vi "Lab Panel V5.26.vi"() -> ()   [LabVIEW 2017] (continued)
                                n855 = TDMS Open(6:FALSE, 10:T21."create or replace" ("operation (0:open)"), 11:w1499) -> (0:w1498:errorcluster, 3:→"TDMS LAB03-2":refnum<k34>)  [unwired: 4 in]
                              }
                              frame #2 {
                                n856 = local read "SET LAB03-2"() -> (w1509:T5)
                                n857 = local read "TDMS LAB03-2"() -> (w1520:refnum<k34>)
                                n858 = Build Array("Testers Name", "Description", "Set Test Cycles", "T-Rise minutes", "T-Rise Deg C") -> (w1510:string[])
                                n859 = Unbundle(w1509) -> ("NAME"=w1508:string, "DESCRIPTION"=w1507:string, "CYCLES"=w1506:dbl, "T-RISE mins"=w1505:dbl, "T-RISE deg C"=w1504:dbl)
                                n860 = Number To Decimal String(number=w1506) -> (decimal integer string=w1519:string)  [unwired: 1 in]
                                n861 = Number To Decimal String(number=w1505) -> (decimal integer string=w1518:string)  [unwired: 1 in]
                                n862 = Number To Decimal String(number=w1504) -> (decimal integer string=w1517:string)  [unwired: 1 in]
                                n863 = Build Array(w1508, w1507, w1519, w1518, w1517) -> (w1516:string[])
                                n864 = TDMS Set Properties(5:w1516, 7:w1510, 11:w1520) -> ()  [unwired: 3 in, 4 out]
                              }
                              frame #3 {
                                n865 = local read "DISP LAB03-2"() -> (w1525:T4)
                                n866 = Concatenate Strings("LAB03-2  ", w1524) -> (w1526:string)
                                n867 = Two Button Dialog(message=w1526, 1:w1522, 2:w1523) -> (T button?=w1528:bool)
                                n868 = case shown="True" w1528 {
                                tunnel: w1525 -> [w1535 w1536]
                                tunnel: [w1535 w1536] -> w1532
                                tunnel: [w1534 w1537] -> w1531
                                tunnel: [w1533 w1537] -> w1530
                                frame False {
                                n869 = Unbundle(w1535) -> ("CYCLE"=w1534:dbl, "MINS"=w1533:dbl)  [unwired: 1 out]
                                }
                                frame True {
                                w1537 = 0.0
                                }
                                }
                                n870 = Bundle(cluster=w1532, "CYCLE"=w1531, "MINS"=w1530, "STATUS"="RUN") -> (w1521:T4)
                                n871 = local write "DISP LAB03-2"(w1521) -> ()
                              }
                              frame #4 {
                                n872 = local read "TEMP START LAB03-2"() -> (w1540:cluster{"TL":dbl, "TN":dbl})
                                n873 = Bundle(cluster=w1540, "TL"=w1538, "TN"=w1538) -> (w1539:cluster{"TL":dbl, "TN":dbl})
                                n874 = local write "TEMP START LAB03-2"(w1539) -> ()
                              }
                            }
                          }
                        }
                      }
                    }
                  }
                }
              }
              event "RUN LAB04-1": Value Change {
                n875 = event-data() -> ("NewVal"=w1545:bool)  [unwired: 1 in, 5 out]
                n876 = local write "run lab04-1"(w1545) -> ()
                n877 = case shown="True" w1545 {
                  tunnel: w1551 -> [_ w1589]
                  tunnel: w1550 -> [_ w1588]
                  tunnel: w1548 -> [w1553 w1587]
                  tunnel: w1549 -> [_ w1586]
                  tunnel: w1547 -> [_ w1585]
                  tunnel: [w1552 w1584] -> w1546
                  tunnel: w1544 -> [_ w1583]
                  tunnel: w1543 -> [_ w1582]
                  tunnel: w1542 -> [_ w1581]
                  tunnel: w1541 -> [_ w1579]
                  frame False {
                    # "stop test"
                    n878 = stacked-sequence {
                      tunnel: w1553 -> [w1562 _]
                      tunnel: [w1554 _] -> w1552
                      frame #0 {
                        n879 = local read "DISP LAB04-1"() -> (w1561:T4)
                        n880 = Unbundle(w1561) -> ("CYCLE"=w1559:dbl, "MINS"=w1560:dbl)  [unwired: 1 out]
                        n881 = case shown="\"CYCLE TEST\"" w1562 {
                          tunnel: w1560 -> [_ _ w1569]
                          tunnel: w1559 -> [w1567 w1568 _]
                          tunnel: [w1567 w1568 w1569] -> w1558
                          frame "CHART TEST", Default {
                          }
                          frame "CYCLE TEST" {
                          }
                          frame "T-RISE TEST" {
                          }
                        }
                        n882 = local read "TDMS LAB04-1"() -> (w1566:refnum<k34>)
                        n883 = Build Array("STOPPED") -> (w1563:string[])
                        n884 = Build Array(w1558) -> (w1557:dbl[])
                        n885 = TDMS Write(0:w1566, 5:"TEST RESULT", 7:w1563, 9:w1557) -> (4:w1555:refnum<k34>, 15:w1556:errorcluster)  [unwired: 2 in, 2 out]
                        n886 = TDMS Close(8:w1556, 11:w1555) -> (0:w1554:errorcluster)  [unwired: 1 out]
                      }
                      frame #1 {
                        n887 = local read "DISP LAB04-1"() -> (w1573:T4)
                        n888 = stacked-sequence {
                          tunnel: "LAB04-1" -> [w1575 w1577]
                          frame #0 {
                            n889 = call "sub vi - defrag tdms v1.vi"("panel id"=w1575) -> ("error out"=w1574:errorcluster)  [unwired: 10 in]
                            n890 = local write "data file error"(w1574) -> ()
                          }
                          frame #1 {
                            n891 = call "Save data file (stop) v3.vi"("panel id"=w1577) -> ("network file save error"=w1576:errorcluster)  [unwired: 9 in, 1 out]
                            n892 = local write "RESULT LAB04-1"(FALSE) -> ()
                            n893 = local write "data file error"(w1576) -> ()
                          }
                        }
                        n894 = Bundle(cluster=w1573, "STATUS"="STOP") -> (w1571:T4)  [unwired: 2 in]
                        n895 = local write "DISP LAB04-1"(w1571) -> ()
                      }
                    }
                  }
                  frame True {
                    n896 = local read "SIG LAB04-1"() -> (w1580:T2)
                    n897 = stacked-sequence {
                      seq-local: [w1591 _] -> [_ w1595]
                      tunnel: w1589 -> [_ w1605]
                      tunnel: w1588 -> [_ w1604]
                      tunnel: w1587 -> [_ w1603]
                      tunnel: w1586 -> [_ w1602]
                      tunnel: w1585 -> [_ w1601]
                      tunnel: [_ w1600] -> w1584
                      tunnel: w1583 -> [_ w1599]
                      tunnel: w1582 -> [_ w1598]
                      tunnel: w1581 -> [_ w1597]
                      tunnel: w1580 -> [w1590 w1596]
                      tunnel: w1579 -> [_ w1594]
                      frame #0 {
                        n898 = Unbundle(w1590) -> ("AMPS"=w1593:dbl)  [unwired: 4 out]
                        n899 = call "Check For Amps on v1.vi"("ID"="LAB04-1", "amps"=w1593) -> ("amps"=w1591:bool)  [unwired: 9 in]
                      }
                      frame #1 {
                        n900 = case shown="True" w1595 {
                          tunnel: w1605 -> [_ w1618]
                          tunnel: w1604 -> [_ w1617]
                          tunnel: w1603 -> [_ w1616]
                          tunnel: w1602 -> [_ w1615]
                          tunnel: w1601 -> [_ w1614]
                          tunnel: [errorcluster {"status"=FALSE, "code"=0, "source"=""} ("error out") w1613] -> w1600
                          tunnel: w1599 -> [_ w1612]
                          tunnel: w1598 -> [_ w1611]
                          tunnel: w1597 -> [_ w1610]
                          tunnel: w1596 -> [_ w1609]
                          tunnel: w1594 -> [_ w1608]
                          frame False {
                            w1606 = FALSE
                            n901 = local write "RUN LAB04-1"(w1606) -> ()
                            n902 = local write "run lab04-1"(w1606) -> ()
                          }
                          frame True {
                            n903 = stacked-sequence {
                              seq-local: [w1619 _ _ _ _] -> [_ w1643 _ _ _]
                              tunnel: w1618 -> [w1624 _ _ _ _]
                              tunnel: w1617 -> [w1620 _ _ _ _]
                              tunnel: w1616 -> [w1634 _ _ _ _]
                              tunnel: w1615 -> [w1627 _ _ _ _]
                              tunnel: w1614 -> [w1622 _ _ _ _]
                              tunnel: [_ w1638 _ _ _] -> w1613
                              tunnel: w1612 -> [_ _ _ w1664 _]
                              tunnel: w1611 -> [_ _ _ w1663 _]
                              tunnel: w1610 -> [_ _ _ w1662 _]
                              tunnel: w1609 -> [_ _ _ _ _]
                              tunnel: w1608 -> [_ _ _ _ w1678]
                              frame #0 {
                                w1621 = "\\"
                                n904 = local read "SET LAB04-1"() -> (w1629:T5)
                                n905 = case shown="\"CYCLE TEST\"" w1634 {
                                tunnel: ["L04-1-CHART TEST-" "L04-1-CYCLE TEST-" "L04-1-T-RISE TEST-"] -> w1630
                                frame "CHART TEST", Default {
                                }
                                frame "CYCLE TEST" {
                                }
                                frame "T-RISE TEST" {
                                }
                                }
                                n906 = Unbundle(w1629) -> ("DESCRIPTION"=w1628:string)  [unwired: 4 out]
                                n907 = Concatenate Strings(w1624, "\\", w1622, w1621, w1620, w1621) -> (w1631:string)
                                n908 = String To Path(string=w1631) -> (path=w1633:path)
                                n909 = Concatenate Strings(w1631, w1630, w1628, "-", w1627, ".tdms") -> (w1619:string)
                                n910 = Create Folder(path (use dialog)=w1633) -> (error out=w1632:errorcluster)  [unwired: 2 in, 2 out]
                                n911 = global write "Global 1.vi" "LAB04-1 FILE"(w1619) -> ()
                                n912 = call <vilib>:"Clear Errors.vi"("error in (no error)"=w1632) -> ()  [unwired: 5 in, 2 out]
                              }
                              frame #1 {
                                (unwired) FALSE
                                n913 = String To Path(string=w1643) -> (path=w1639:path)
                                n914 = TDMS Open(6:FALSE, 10:T21."create or replace" ("operation (0:open)"), 11:w1639) -> (0:w1638:errorcluster, 3:→"TDMS LAB04-1":refnum<k34>)  [unwired: 4 in]
                              }
                              frame #2 {
                                n915 = local read "SET LAB04-1"() -> (w1649:T5)
                                n916 = local read "TDMS LAB04-1"() -> (w1660:refnum<k34>)
                                n917 = Build Array("Testers Name", "Description", "Set Test Cycles", "T-Rise minutes", "T-Rise Deg C") -> (w1650:string[])
                                n918 = Unbundle(w1649) -> ("NAME"=w1648:string, "DESCRIPTION"=w1647:string, "CYCLES"=w1646:dbl, "T-RISE mins"=w1645:dbl, "T-RISE deg C"=w1644:dbl)
                                n919 = Number To Decimal String(number=w1646) -> (decimal integer string=w1659:string)  [unwired: 1 in]
                                n920 = Number To Decimal String(number=w1645) -> (decimal integer string=w1658:string)  [unwired: 1 in]
                                n921 = Number To Decimal String(number=w1644) -> (decimal integer string=w1657:string)  [unwired: 1 in]
                                n922 = Build Array(w1648, w1647, w1659, w1658, w1657) -> (w1656:string[])
                                n923 = TDMS Set Properties(5:w1656, 7:w1650, 11:w1660) -> ()  [unwired: 3 in, 4 out]
                              }
                              frame #3 {
                                n924 = local read "DISP LAB04-1"() -> (w1665:T4)
                                n925 = Concatenate Strings("LAB04-1  ", w1664) -> (w1666:string)
                                n926 = Two Button Dialog(message=w1666, 1:w1662, 2:w1663) -> (T button?=w1668:bool)
                                n927 = case shown="True" w1668 {
                                tunnel: w1665 -> [w1675 w1676]
                                tunnel: [w1675 w1676] -> w1672
                                tunnel: [w1674 w1677] -> w1671
                                tunnel: [w1673 w1677] -> w1670
                                frame False {
                                n928 = Unbundle(w1675) -> ("CYCLE"=w1674:dbl, "MINS"=w1673:dbl)  [unwired: 1 out]
                                }
                                frame True {
                                w1677 = 0.0
                                }
                                }
                                n929 = Bundle(cluster=w1672, "CYCLE"=w1671, "MINS"=w1670, "STATUS"="RUN") -> (w1661:T4)
                                n930 = local write "DISP LAB04-1"(w1661) -> ()
                              }
                              frame #4 {
                                n931 = local read "TEMP START LAB04-1"() -> (w1680:cluster{"TL":dbl, "TN":dbl})
                                n932 = Bundle(cluster=w1680, "TL"=w1678, "TN"=w1678) -> (w1679:cluster{"TL":dbl, "TN":dbl})
                                n933 = local write "TEMP START LAB04-1"(w1679) -> ()
                              }
                            }
                          }
                        }
                      }
                    }
                  }
                }
              }
              event "RUN LAB04-2": Value Change {
                n934 = event-data() -> ("NewVal"=w1685:bool)  [unwired: 1 in, 5 out]
                n935 = local write "run lab04-2"(w1685) -> ()
                n936 = case shown="True" w1685 {
                  tunnel: w1691 -> [_ w1729]
                  tunnel: w1690 -> [_ w1728]
                  tunnel: w1688 -> [w1693 w1727]
                  tunnel: w1689 -> [_ w1726]
                  tunnel: w1687 -> [_ w1725]
                  tunnel: [w1692 w1724] -> w1686
                  tunnel: w1684 -> [_ w1723]
                  tunnel: w1683 -> [_ w1722]
                  tunnel: w1682 -> [_ w1721]
                  tunnel: w1681 -> [_ w1719]
                  frame False {
                    # "stop test"
                    n937 = stacked-sequence {
                      tunnel: w1693 -> [w1702 _]
                      tunnel: [w1694 _] -> w1692
                      frame #0 {
                        n938 = local read "DISP LAB04-2"() -> (w1701:T4)
                        n939 = Unbundle(w1701) -> ("CYCLE"=w1699:dbl, "MINS"=w1700:dbl)  [unwired: 1 out]
                        n940 = case shown="\"CYCLE TEST\"" w1702 {
                          tunnel: w1700 -> [_ _ w1709]
                          tunnel: w1699 -> [w1707 w1708 _]
                          tunnel: [w1707 w1708 w1709] -> w1698
                          frame "CHART TEST", Default {
                          }
                          frame "CYCLE TEST" {
                          }
                          frame "T-RISE TEST" {
                          }
                        }
                        n941 = local read "TDMS LAB04-2"() -> (w1706:refnum<k34>)
                        n942 = Build Array("STOPPED") -> (w1703:string[])
                        n943 = Build Array(w1698) -> (w1697:dbl[])
                        n944 = TDMS Write(0:w1706, 5:"TEST RESULT", 7:w1703, 9:w1697) -> (4:w1695:refnum<k34>, 15:w1696:errorcluster)  [unwired: 2 in, 2 out]
                        n945 = TDMS Close(8:w1696, 11:w1695) -> (0:w1694:errorcluster)  [unwired: 1 out]
                      }
                      frame #1 {
                        n946 = local read "DISP LAB04-2"() -> (w1713:T4)
                        n947 = stacked-sequence {
                          tunnel: "LAB04-2" -> [w1715 w1717]
                          frame #0 {
                            n948 = call "sub vi - defrag tdms v1.vi"("panel id"=w1715) -> ("error out"=w1714:errorcluster)  [unwired: 10 in]
                            n949 = local write "data file error"(w1714) -> ()
                          }
                          frame #1 {
                            n950 = call "Save data file (stop) v3.vi"("panel id"=w1717) -> ("network file save error"=w1716:errorcluster)  [unwired: 9 in, 1 out]
                            n951 = local write "RESULT LAB04-2"(FALSE) -> ()
                            n952 = local write "data file error"(w1716) -> ()
                          }
                        }
                        n953 = Bundle(cluster=w1713, "STATUS"="STOP") -> (w1711:T4)  [unwired: 2 in]
                        n954 = local write "DISP LAB04-2"(w1711) -> ()
                      }
                    }
                  }
                  frame True {
                    n955 = local read "SIG LAB04-2"() -> (w1720:T2)
                    n956 = stacked-sequence {
                      seq-local: [w1731 _] -> [_ w1735]
                      tunnel: w1729 -> [_ w1745]
                      tunnel: w1728 -> [_ w1744]
                      tunnel: w1727 -> [_ w1743]
                      tunnel: w1726 -> [_ w1742]
                      tunnel: w1725 -> [_ w1741]
                      tunnel: [_ w1740] -> w1724
                      tunnel: w1723 -> [_ w1739]
                      tunnel: w1722 -> [_ w1738]
                      tunnel: w1721 -> [_ w1737]
                      tunnel: w1720 -> [w1730 w1736]
                      tunnel: w1719 -> [_ w1734]
                      frame #0 {
                        n957 = Unbundle(w1730) -> ("AMPS"=w1733:dbl)  [unwired: 4 out]
                        n958 = call "Check For Amps on v1.vi"("ID"="LAB04-2", "amps"=w1733) -> ("amps"=w1731:bool)  [unwired: 9 in]
                      }
                      frame #1 {
                        n959 = case shown="True" w1735 {
                          tunnel: w1745 -> [_ w1758]
                          tunnel: w1744 -> [_ w1757]
                          tunnel: w1743 -> [_ w1756]
                          tunnel: w1742 -> [_ w1755]
                          tunnel: w1741 -> [_ w1754]
                          tunnel: [errorcluster {"status"=FALSE, "code"=0, "source"=""} ("error out") w1753] -> w1740
                          tunnel: w1739 -> [_ w1752]
                          tunnel: w1738 -> [_ w1751]
                          tunnel: w1737 -> [_ w1750]
                          tunnel: w1736 -> [_ w1749]
                          tunnel: w1734 -> [_ w1748]
                          frame False {
                            w1746 = FALSE
                            n960 = local write "RUN LAB04-2"(w1746) -> ()
                            n961 = local write "run lab04-2"(w1746) -> ()
                          }
                          frame True {
                            n962 = stacked-sequence {
                              seq-local: [w1759 _ _ _ _] -> [_ w1783 _ _ _]
                              tunnel: w1758 -> [w1764 _ _ _ _]
                              tunnel: w1757 -> [w1760 _ _ _ _]
                              tunnel: w1756 -> [w1774 _ _ _ _]
                              tunnel: w1755 -> [w1767 _ _ _ _]
                              tunnel: w1754 -> [w1762 _ _ _ _]
                              tunnel: [_ w1778 _ _ _] -> w1753
                              tunnel: w1752 -> [_ _ _ w1804 _]
                              tunnel: w1751 -> [_ _ _ w1803 _]
                              tunnel: w1750 -> [_ _ _ w1802 _]
                              tunnel: w1749 -> [_ _ _ _ _]
                              tunnel: w1748 -> [_ _ _ _ w1818]
                              frame #0 {
                                w1761 = "\\"
                                n963 = local read "SET LAB04-2"() -> (w1769:T5)
                                n964 = case shown="\"CHART TEST\", Default" w1774 {
                                tunnel: ["L04-2-CHART TEST-" "L04-2-CYCLE TEST-" "L04-2-T-RISE TEST-"] -> w1770
                                frame "CHART TEST", Default {
                                }
                                frame "CYCLE TEST" {
                                }
                                frame "T-RISE TEST" {
                                }
                                }
                                n965 = Unbundle(w1769) -> ("DESCRIPTION"=w1768:string)  [unwired: 4 out]
                                n966 = Concatenate Strings(w1764, "\\", w1762, w1761, w1760, w1761) -> (w1771:string)
                                n967 = String To Path(string=w1771) -> (path=w1773:path)
                                n968 = Concatenate Strings(w1771, w1770, w1768, "-", w1767, ".tdms") -> (w1759:string)
                                n969 = Create Folder(path (use dialog)=w1773) -> (error out=w1772:errorcluster)  [unwired: 2 in, 2 out]
                                n970 = global write "Global 1.vi" "LAB04-2 FILE"(w1759) -> ()
                                n971 = call <vilib>:"Clear Errors.vi"("error in (no error)"=w1772) -> ()  [unwired: 5 in, 2 out]
                              }
                              frame #1 {
                                (unwired) FALSE
                                n972 = String To Path(string=w1783) -> (path=w1779:path)
                                n973 = TDMS Open(6:FALSE, 10:T21."create or replace" ("operation (0:open)"), 11:w1779) -> (0:w1778:errorcluster, 3:→"TDMS LAB04-2":refnum<k34>)  [unwired: 4 in]
                              }
                              frame #2 {
                                n974 = local read "SET LAB04-2"() -> (w1789:T5)
                                n975 = local read "TDMS LAB04-2"() -> (w1800:refnum<k34>)
                                n976 = Build Array("Testers Name", "Description", "Set Test Cycles", "T-Rise minutes", "T-Rise Deg C") -> (w1790:string[])
                                n977 = Unbundle(w1789) -> ("NAME"=w1788:string, "DESCRIPTION"=w1787:string, "CYCLES"=w1786:dbl, "T-RISE mins"=w1785:dbl, "T-RISE deg C"=w1784:dbl)
                                n978 = Number To Decimal String(number=w1786) -> (decimal integer string=w1799:string)  [unwired: 1 in]
                                n979 = Number To Decimal String(number=w1785) -> (decimal integer string=w1798:string)  [unwired: 1 in]
                                n980 = Number To Decimal String(number=w1784) -> (decimal integer string=w1797:string)  [unwired: 1 in]
                                n981 = Build Array(w1788, w1787, w1799, w1798, w1797) -> (w1796:string[])
                                n982 = TDMS Set Properties(5:w1796, 7:w1790, 11:w1800) -> ()  [unwired: 3 in, 4 out]
                              }
                              frame #3 {
                                n983 = local read "DISP LAB04-2"() -> (w1805:T4)
                                n984 = Concatenate Strings("LAB04-2 ", w1804) -> (w1806:string)
                                n985 = Two Button Dialog(message=w1806, 1:w1802, 2:w1803) -> (T button?=w1808:bool)
                                n986 = case shown="True" w1808 {
                                tunnel: w1805 -> [w1815 w1816]
                                tunnel: [w1815 w1816] -> w1812
                                tunnel: [w1814 w1817] -> w1811
                                tunnel: [w1813 w1817] -> w1810
                                frame False {
                                n987 = Unbundle(w1815) -> ("CYCLE"=w1814:dbl, "MINS"=w1813:dbl)  [unwired: 1 out]
                                }
                                frame True {
                                w1817 = 0.0
                                }
                                }
                                n988 = Bundle(cluster=w1812, "CYCLE"=w1811, "MINS"=w1810, "STATUS"="RUN") -> (w1801:T4)
                                n989 = local write "DISP LAB04-2"(w1801) -> ()
                              }
                              frame #4 {
                                n990 = local read "TEMP START LAB04-2"() -> (w1820:cluster{"TL":dbl, "TN":dbl})
                                n991 = Bundle(cluster=w1820, "TL"=w1818, "TN"=w1818) -> (w1819:cluster{"TL":dbl, "TN":dbl})
                                n992 = local write "TEMP START LAB04-2"(w1819) -> ()
                              }
                            }
                          }
                        }
                      }
                    }
                  }
                }
              }
              event "RUN LAB05-1": Value Change {
                n993 = event-data() -> ("NewVal"=w1825:bool)  [unwired: 1 in, 5 out]
                n994 = local write "run lab05-1"(w1825) -> ()
                n995 = case shown="True" w1825 {
                  tunnel: w1831 -> [_ w1869]
                  tunnel: w1830 -> [_ w1868]
                  tunnel: w1828 -> [w1833 w1867]
                  tunnel: w1829 -> [_ w1866]
                  tunnel: w1827 -> [_ w1865]
                  tunnel: [w1832 w1864] -> w1826
                  tunnel: w1824 -> [_ w1863]
                  tunnel: w1823 -> [_ w1862]
                  tunnel: w1822 -> [_ w1861]
                  tunnel: w1821 -> [_ w1859]
                  frame False {
                    # "stop test"
                    n996 = stacked-sequence {
                      tunnel: w1833 -> [w1842 _]
                      tunnel: [w1834 _] -> w1832
                      frame #0 {
                        n997 = local read "DISP LAB05-1"() -> (w1841:T4)
                        n998 = Unbundle(w1841) -> ("CYCLE"=w1839:dbl, "MINS"=w1840:dbl)  [unwired: 1 out]
                        n999 = case shown="\"CYCLE TEST\"" w1842 {
                          tunnel: w1840 -> [_ _ w1849]
                          tunnel: w1839 -> [w1847 w1848 _]
                          tunnel: [w1847 w1848 w1849] -> w1838
                          frame "CHART TEST", Default {
                          }
                          frame "CYCLE TEST" {
                          }
                          frame "T-RISE TEST" {
                          }
                        }
                        n1000 = local read "TDMS LAB05-1"() -> (w1846:refnum<k34>)
                        n1001 = Build Array("STOPPED") -> (w1843:string[])
                        n1002 = Build Array(w1838) -> (w1837:dbl[])
                        n1003 = TDMS Write(0:w1846, 5:"TEST RESULT", 7:w1843, 9:w1837) -> (4:w1835:refnum<k34>, 15:w1836:errorcluster)  [unwired: 2 in, 2 out]
                        n1004 = TDMS Close(8:w1836, 11:w1835) -> (0:w1834:errorcluster)  [unwired: 1 out]
                      }
                      frame #1 {
                        n1005 = local read "DISP LAB05-1"() -> (w1853:T4)
                        n1006 = stacked-sequence {
                          tunnel: "LAB05-1" -> [w1855 w1857]
                          frame #0 {
                            n1007 = call "sub vi - defrag tdms v1.vi"("panel id"=w1855) -> ("error out"=w1854:errorcluster)  [unwired: 10 in]
                            n1008 = local write "data file error"(w1854) -> ()
                          }
                          frame #1 {
                            n1009 = call "Save data file (stop) v3.vi"("panel id"=w1857) -> ("network file save error"=w1856:errorcluster)  [unwired: 9 in, 1 out]
                            n1010 = local write "RESULT LAB05-1"(FALSE) -> ()
                            n1011 = local write "data file error"(w1856) -> ()
                          }
                        }
                        n1012 = Bundle(cluster=w1853, "STATUS"="STOP") -> (w1851:T4)  [unwired: 2 in]
                        n1013 = local write "DISP LAB05-1"(w1851) -> ()
                      }
                    }
                  }
                  frame True {
                    n1014 = local read "SIG LAB05-1"() -> (w1860:T2)
                    n1015 = stacked-sequence {
                      seq-local: [w1871 _] -> [_ w1875]
                      tunnel: w1869 -> [_ w1885]
                      tunnel: w1868 -> [_ w1884]
                      tunnel: w1867 -> [_ w1883]
                      tunnel: w1866 -> [_ w1882]
                      tunnel: w1865 -> [_ w1881]
                      tunnel: [_ w1880] -> w1864
                      tunnel: w1863 -> [_ w1879]
                      tunnel: w1862 -> [_ w1878]
                      tunnel: w1861 -> [_ w1877]
                      tunnel: w1860 -> [w1870 w1876]
                      tunnel: w1859 -> [_ w1874]
                      frame #0 {
                        n1016 = Unbundle(w1870) -> ("AMPS"=w1873:dbl)  [unwired: 4 out]
                        n1017 = call "Check For Amps on v1.vi"("ID"="LAB05-1", "amps"=w1873) -> ("amps"=w1871:bool)  [unwired: 9 in]
                      }
                      frame #1 {
                        n1018 = case shown="True" w1875 {
                          tunnel: w1885 -> [_ w1898]
                          tunnel: w1884 -> [_ w1897]
                          tunnel: w1883 -> [_ w1896]
                          tunnel: w1882 -> [_ w1895]
                          tunnel: w1881 -> [_ w1894]
                          tunnel: [errorcluster {"status"=FALSE, "code"=0, "source"=""} ("error out") w1893] -> w1880
                          tunnel: w1879 -> [_ w1892]
                          tunnel: w1878 -> [_ w1891]
                          tunnel: w1877 -> [_ w1890]
                          tunnel: w1876 -> [_ w1889]
                          tunnel: w1874 -> [_ w1888]
                          frame False {
                            w1886 = FALSE
                            n1019 = local write "RUN LAB05-1"(w1886) -> ()
                            n1020 = local write "run lab05-1"(w1886) -> ()
                          }
                          frame True {
                            n1021 = stacked-sequence {
                              seq-local: [w1899 _ _ _ _] -> [_ w1923 _ _ _]
                              tunnel: w1898 -> [w1904 _ _ _ _]
                              tunnel: w1897 -> [w1900 _ _ _ _]
                              tunnel: w1896 -> [w1914 _ _ _ _]
                              tunnel: w1895 -> [w1907 _ _ _ _]
                              tunnel: w1894 -> [w1902 _ _ _ _]
                              tunnel: [_ w1918 _ _ _] -> w1893
                              tunnel: w1892 -> [_ _ _ w1943 _]
                              tunnel: w1891 -> [_ _ _ w1942 _]
                              tunnel: w1890 -> [_ _ _ w1941 _]
                              tunnel: w1889 -> [_ _ _ _ _]
                              tunnel: w1888 -> [_ _ _ _ w1958]
                              frame #0 {
                                w1901 = "\\"
                                n1022 = local read "SET LAB05-1"() -> (w1909:T5)
                                n1023 = case shown="\"CYCLE TEST\"" w1914 {
                                tunnel: ["L05-1-CHART TEST-" "L05-1-CYCLE TEST-" "L05-1-T-RISE TEST-"] -> w1910
                                frame "CHART TEST", Default {
                                }
                                frame "CYCLE TEST" {
                                }
                                frame "T-RISE TEST" {
                                }
                                }
                                n1024 = Unbundle(w1909) -> ("DESCRIPTION"=w1908:string)  [unwired: 4 out]
                                n1025 = Concatenate Strings(w1904, "\\", w1902, w1901, w1900, w1901) -> (w1911:string)
                                n1026 = String To Path(string=w1911) -> (path=w1913:path)
                                n1027 = Concatenate Strings(w1911, w1910, w1908, "-", w1907, ".tdms") -> (w1899:string)
                                n1028 = Create Folder(path (use dialog)=w1913) -> (error out=w1912:errorcluster)  [unwired: 2 in, 2 out]
                                n1029 = global write "Global 1.vi" "LAB05-1 FILE"(w1899) -> ()
                                n1030 = call <vilib>:"Clear Errors.vi"("error in (no error)"=w1912) -> ()  [unwired: 5 in, 2 out]
                              }
                              frame #1 {
                                (unwired) FALSE
                                n1031 = String To Path(string=w1923) -> (path=w1919:path)
                                n1032 = TDMS Open(6:FALSE, 10:T21."create or replace" ("operation (0:open)"), 11:w1919) -> (0:w1918:errorcluster, 3:→"TDMS LAB05-1":refnum<k34>)  [unwired: 4 in]
                              }
                              frame #2 {
                                n1033 = local read "SET LAB05-1"() -> (w1929:T5)
                                n1034 = local read "TDMS LAB05-1"() -> (w1940:refnum<k34>)
                                n1035 = Build Array("Testers Name", "Description", "Set Test Cycles", "T-Rise minutes", "T-Rise Deg C") -> (w1930:string[])
                                n1036 = Unbundle(w1929) -> ("NAME"=w1928:string, "DESCRIPTION"=w1927:string, "CYCLES"=w1926:dbl, "T-RISE mins"=w1925:dbl, "T-RISE deg C"=w1924:dbl)
                                n1037 = Number To Decimal String(number=w1926) -> (decimal integer string=w1939:string)  [unwired: 1 in]
                                n1038 = Number To Decimal String(number=w1925) -> (decimal integer string=w1938:string)  [unwired: 1 in]
                                n1039 = Number To Decimal String(number=w1924) -> (decimal integer string=w1937:string)  [unwired: 1 in]
                                n1040 = Build Array(w1928, w1927, w1939, w1938, w1937) -> (w1936:string[])
                                n1041 = TDMS Set Properties(5:w1936, 7:w1930, 11:w1940) -> ()  [unwired: 3 in, 4 out]
                              }
                              frame #3 {
                                n1042 = local read "DISP LAB05-1"() -> (w1945:T4)
                                n1043 = Concatenate Strings("LAB05-1  ", w1943) -> (w1946:string)
                                n1044 = Two Button Dialog(message=w1946, 1:w1941, 2:w1942) -> (T button?=w1948:bool)
                                n1045 = case shown="True" w1948 {
                                tunnel: w1945 -> [w1955 w1956]
                                tunnel: [w1955 w1956] -> w1952
                                tunnel: [w1954 w1957] -> w1951
                                tunnel: [w1953 w1957] -> w1950
                                frame False {
                                n1046 = Unbundle(w1955) -> ("CYCLE"=w1954:dbl, "MINS"=w1953:dbl)  [unwired: 1 out]
                                }
                                frame True {
                                w1957 = 0.0
                                }
                                }
                                n1047 = Bundle(cluster=w1952, "CYCLE"=w1951, "MINS"=w1950, "STATUS"="RUN") -> (w1944:T4)
                                n1048 = local write "DISP LAB05-1"(w1944) -> ()
                              }
                              frame #4 {
                                n1049 = local read "TEMP START LAB05-1"() -> (w1960:cluster{"TL":dbl, "TN":dbl})
                                n1050 = Bundle(cluster=w1960, "TL"=w1958, "TN"=w1958) -> (w1959:cluster{"TL":dbl, "TN":dbl})
                                n1051 = local write "TEMP START LAB05-1"(w1959) -> ()
                              }
                            }
                          }
                        }
                      }
                    }
                  }
                }
              }
              event "RUN LAB05-2": Value Change {
                n1052 = event-data() -> ("NewVal"=w1966:bool)  [unwired: 1 in, 5 out]
                n1053 = local read "SIG LAB05-2"() -> (w1962:T2)
                n1054 = case shown="True" w1966 {
                  tunnel: w1972 -> [_ w2010]
                  tunnel: w1971 -> [_ w2009]
                  tunnel: w1969 -> [w1974 w2008]
                  tunnel: w1970 -> [_ w2007]
                  tunnel: w1968 -> [_ w2006]
                  tunnel: [w1973 w2005] -> w1967
                  tunnel: w1965 -> [_ w2004]
                  tunnel: w1964 -> [_ w2003]
                  tunnel: w1963 -> [_ w2002]
                  tunnel: w1962 -> [_ w2001]
                  tunnel: w1961 -> [_ w2000]
                  frame False {
                    # "stop test"
                    n1055 = stacked-sequence {
                      tunnel: w1974 -> [w1983 _]
                      tunnel: [w1975 _] -> w1973
                      frame #0 {
                        n1056 = local read "DISP LAB05-2"() -> (w1982:T4)
                        n1057 = Unbundle(w1982) -> ("CYCLE"=w1980:dbl, "MINS"=w1981:dbl)  [unwired: 1 out]
                        n1058 = case shown="\"CYCLE TEST\"" w1983 {
                          tunnel: w1981 -> [_ _ w1990]
                          tunnel: w1980 -> [w1988 w1989 _]
                          tunnel: [w1988 w1989 w1990] -> w1979
                          frame "CHART TEST", Default {
                          }
                          frame "CYCLE TEST" {
                          }
                          frame "T-RISE TEST" {
                          }
                        }
                        n1059 = local read "TDMS LAB05-2"() -> (w1987:refnum<k34>)
                        n1060 = Build Array("STOPPED") -> (w1984:string[])
                        n1061 = Build Array(w1979) -> (w1978:dbl[])
                        n1062 = TDMS Write(0:w1987, 5:"TEST RESULT", 7:w1984, 9:w1978) -> (4:w1976:refnum<k34>, 15:w1977:errorcluster)  [unwired: 2 in, 2 out]
                        n1063 = TDMS Close(8:w1977, 11:w1976) -> (0:w1975:errorcluster)  [unwired: 1 out]
                      }
                      frame #1 {
                        n1064 = local read "DISP LAB05-2"() -> (w1994:T4)
                        n1065 = stacked-sequence {
                          tunnel: "LAB05-2" -> [w1996 w1998]
                          frame #0 {
                            n1066 = call "sub vi - defrag tdms v1.vi"("panel id"=w1996) -> ("error out"=w1995:errorcluster)  [unwired: 10 in]
                            n1067 = local write "data file error"(w1995) -> ()
                          }
                          frame #1 {
                            n1068 = local write "RESULT LAB05-2"(FALSE) -> ()
                            n1069 = call "Save data file (stop) v3.vi"("panel id"=w1998) -> ("network file save error"=w1997:errorcluster)  [unwired: 9 in, 1 out]
                            n1070 = local write "data file error"(w1997) -> ()
                          }
                        }
                        n1071 = Bundle(cluster=w1994, "STATUS"="STOP") -> (w1992:T4)  [unwired: 2 in]
                        n1072 = local write "DISP LAB05-2"(w1992) -> ()
                      }
                    }
                  }
                  frame True {
                    n1073 = stacked-sequence {
                      seq-local: [w2012 _] -> [_ w2016]
                      tunnel: w2010 -> [_ w2026]
                      tunnel: w2009 -> [_ w2025]
                      tunnel: w2008 -> [_ w2024]
                      tunnel: w2007 -> [_ w2023]
                      tunnel: w2006 -> [_ w2022]
                      tunnel: [_ w2021] -> w2005
                      tunnel: w2004 -> [_ w2020]
                      tunnel: w2003 -> [_ w2019]
                      tunnel: w2002 -> [_ w2018]
                      tunnel: w2001 -> [w2011 w2017]
                      tunnel: w2000 -> [_ w2015]
                      frame #0 {
                        n1074 = Unbundle(w2011) -> ("AMPS"=w2014:dbl)  [unwired: 4 out]
                        n1075 = call "Check For Amps on v1.vi"("ID"="LAB05-2", "amps"=w2014) -> ("amps"=w2012:bool)  [unwired: 9 in]
                      }
                      frame #1 {
                        n1076 = case shown="True" w2016 {
                          tunnel: w2026 -> [_ w2039]
                          tunnel: w2025 -> [_ w2038]
                          tunnel: w2024 -> [_ w2037]
                          tunnel: w2023 -> [_ w2036]
                          tunnel: w2022 -> [_ w2035]
                          tunnel: [errorcluster {"status"=FALSE, "code"=0, "source"=""} ("error out") w2034] -> w2021
                          tunnel: w2020 -> [_ w2033]
                          tunnel: w2019 -> [_ w2032]
                          tunnel: w2018 -> [_ w2031]
                          tunnel: w2017 -> [_ w2030]
                          tunnel: w2015 -> [_ w2029]
                          frame False {
                            w2027 = FALSE
                            n1077 = local write "RUN LAB05-2"(w2027) -> ()
                            n1078 = local write "run lab05-2"(w2027) -> ()
                          }
                          frame True {
                            n1079 = stacked-sequence {
                              seq-local: [w2040 _ _ _ _] -> [_ w2064 _ _ _]
                              tunnel: w2039 -> [w2045 _ _ _ _]
                              tunnel: w2038 -> [w2041 _ _ _ _]
                              tunnel: w2037 -> [w2055 _ _ _ _]
                              tunnel: w2036 -> [w2048 _ _ _ _]
                              tunnel: w2035 -> [w2043 _ _ _ _]
                              tunnel: [_ w2059 _ _ _] -> w2034
                              tunnel: w2033 -> [_ _ _ w2084 _]
                              tunnel: w2032 -> [_ _ _ w2083 _]
                              tunnel: w2031 -> [_ _ _ w2082 _]
                              tunnel: w2030 -> [_ _ _ _ _]
                              tunnel: w2029 -> [_ _ _ _ w2099]
                              frame #0 {
                                w2042 = "\\"
                                n1080 = local read "SET LAB05-2"() -> (w2050:T5)
                                n1081 = case shown="\"CYCLE TEST\"" w2055 {
                                tunnel: ["L05-2-CHART TEST-" "L05-2-CYCLE TEST-" "L05-2-T-RISE TEST-"] -> w2051
                                frame "CHART TEST", Default {
                                }
                                frame "CYCLE TEST" {
                                }
                                frame "T-RISE TEST" {
                                }
                                }
                                n1082 = Unbundle(w2050) -> ("DESCRIPTION"=w2049:string)  [unwired: 4 out]
                                n1083 = Concatenate Strings(w2045, "\\", w2043, w2042, w2041, w2042) -> (w2052:string)
                                n1084 = String To Path(string=w2052) -> (path=w2054:path)
                                n1085 = Concatenate Strings(w2052, w2051, w2049, "-", w2048, ".tdms") -> (w2040:string)
                                n1086 = Create Folder(path (use dialog)=w2054) -> (error out=w2053:errorcluster)  [unwired: 2 in, 2 out]
                                n1087 = global write "Global 1.vi" "LAB05-2 FILE"(w2040) -> ()
                                n1088 = call <vilib>:"Clear Errors.vi"("error in (no error)"=w2053) -> ()  [unwired: 5 in, 2 out]
                              }
                              frame #1 {
                                (unwired) FALSE
                                n1089 = String To Path(string=w2064) -> (path=w2060:path)
                                n1090 = TDMS Open(6:FALSE, 10:T21."create or replace" ("operation (0:open)"), 11:w2060) -> (0:w2059:errorcluster, 3:→"TDMS LAB05-2":refnum<k34>)  [unwired: 4 in]
                              }
                              frame #2 {
                                n1091 = local read "SET LAB05-2"() -> (w2070:T5)
                                n1092 = local read "TDMS LAB05-2"() -> (w2081:refnum<k34>)
                                n1093 = Build Array("Testers Name", "Description", "Set Test Cycles", "T-Rise minutes", "T-Rise Deg C") -> (w2071:string[])
                                n1094 = Unbundle(w2070) -> ("NAME"=w2069:string, "DESCRIPTION"=w2068:string, "CYCLES"=w2067:dbl, "T-RISE mins"=w2066:dbl, "T-RISE deg C"=w2065:dbl)
                                n1095 = Number To Decimal String(number=w2067) -> (decimal integer string=w2080:string)  [unwired: 1 in]
                                n1096 = Number To Decimal String(number=w2066) -> (decimal integer string=w2079:string)  [unwired: 1 in]
                                n1097 = Number To Decimal String(number=w2065) -> (decimal integer string=w2078:string)  [unwired: 1 in]
                                n1098 = Build Array(w2069, w2068, w2080, w2079, w2078) -> (w2077:string[])
                                n1099 = TDMS Set Properties(5:w2077, 7:w2071, 11:w2081) -> ()  [unwired: 3 in, 4 out]
                              }
                              frame #3 {
                                n1100 = local read "DISP LAB05-2"() -> (w2086:T4)
                                n1101 = Concatenate Strings("LAB05-2  ", w2084) -> (w2087:string)
                                n1102 = Two Button Dialog(message=w2087, 1:w2082, 2:w2083) -> (T button?=w2089:bool)
                                n1103 = case shown="True" w2089 {
                                tunnel: w2086 -> [w2096 w2097]
                                tunnel: [w2096 w2097] -> w2093
                                tunnel: [w2095 w2098] -> w2092
                                tunnel: [w2094 w2098] -> w2091
                                frame False {
                                n1104 = Unbundle(w2096) -> ("CYCLE"=w2095:dbl, "MINS"=w2094:dbl)  [unwired: 1 out]
                                }
                                frame True {
                                w2098 = 0.0
                                }
                                }
                                n1105 = Bundle(cluster=w2093, "CYCLE"=w2092, "MINS"=w2091, "STATUS"="RUN") -> (w2085:T4)
                                n1106 = local write "DISP LAB05-2"(w2085) -> ()
                              }
                              frame #4 {
                                n1107 = local read "TEMP START LAB05-2"() -> (w2101:cluster{"TL":dbl, "TN":dbl})
                                n1108 = Bundle(cluster=w2101, "TL"=w2099, "TN"=w2099) -> (w2100:cluster{"TL":dbl, "TN":dbl})
                                n1109 = local write "TEMP START LAB05-2"(w2100) -> ()
                              }
                            }
                          }
                        }
                      }
                    }
                  }
                }
                n1110 = local write "run lab05-2"(w1966) -> ()
              }
            }
            n1111 = local write "data file error"(w670) -> ()
          }
          frame #5 {
            # "check if test cycles reached for cycle tests, if so then test pass"
            n1112 = stacked-sequence {
              tunnel: w2121 -> [_ _ _ _ _ _ _ _ _ _]
              tunnel: w2120 -> [_ _ _ _ _ _ _ _ _ _]
              tunnel: w2119 -> [_ _ _ _ _ _ _ _ _ _]
              tunnel: w2118 -> [_ _ _ _ _ _ _ _ _ _]
              tunnel: w2117 -> [_ _ _ _ _ _ _ _ _ _]
              tunnel: w2116 -> [_ _ _ _ _ _ _ _ _ _]
              tunnel: w2115 -> [_ _ _ _ _ _ _ _ _ _]
              tunnel: w2114 -> [_ _ _ _ _ _ _ _ _ _]
              tunnel: w2113 -> [_ _ _ _ _ _ _ _ _ _]
              tunnel: w2112 -> [_ _ _ _ _ _ _ _ _ _]
              tunnel: w2111 -> [w2127 _ _ _ _ _ _ _ _ _]
              tunnel: w2110 -> [_ w2162 _ _ _ _ _ _ _ _]
              tunnel: w2109 -> [_ _ w2202 _ _ _ _ _ _ _]
              tunnel: w2108 -> [_ _ _ w2242 _ _ _ _ _ _]
              tunnel: w2107 -> [_ _ _ _ w2282 _ _ _ _ _]
              tunnel: w2106 -> [_ _ _ _ _ w2322 _ _ _ _]
              tunnel: w2105 -> [_ _ _ _ _ _ w2362 _ _ _]
              tunnel: w2104 -> [_ _ _ _ _ _ _ w2402 _ _]
              tunnel: w2103 -> [_ _ _ _ _ _ _ _ w2442 _]
              tunnel: w2102 -> [_ _ _ _ _ _ _ _ _ w2482]
              frame #0 {
                # "LAB01-1"
                n1113 = Less?(x=w2127, y=2) -> (x < y?=w2125:bool)
                n1114 = local read "DISP LAB01-1"() -> (w2128:T4)
                n1115 = Unbundle(w2128) -> ("STATUS"=w2122:string)  [unwired: 2 out]
                n1116 = Equal?(x=w2122, y="RUN") -> (x = y?=w2124:bool)
                n1117 = And(x=w2124, y=w2125) -> (x .and. y?=w2123:bool)
                n1118 = case shown="True" w2123 {
                  tunnel: w2128 -> [_ w2133]
                  tunnel: w2127 -> [_ w2137]
                  frame False {
                  }
                  frame True {
                    n1119 = local read "SET LAB01-1"() -> (w2139:T5)
                    n1120 = local read "TDMS LAB01-1"() -> (w2132:refnum<k34>)
                    n1121 = Unbundle(w2139) -> ("CYCLES"=w2130:dbl, "T-RISE mins"=w2136:dbl)  [unwired: 3 out]
                    n1122 = case shown="\"CYCLE TEST\"" w2137 {
                      tunnel: w2136 -> [_ _ w2146]
                      tunnel: [w2141 w2143 w2146] -> w2135
                      tunnel: w2130 -> [w2141 w2143 _]
                      tunnel: ["CHART PASS" "CYCLE PASS" "T-RISE PASS"] -> w2134
                      frame "CHART TEST", Default {
                      }
                      frame "CYCLE TEST" {
                      }
                      frame "T-RISE TEST" {
                      }
                    }
                    n1123 = Unbundle(w2133) -> ("CYCLE"=w2138:dbl)  [unwired: 2 out]
                    n1124 = Increment(x=w2130) -> (x+1=w2131:dbl)
